vi "Driver Init.vi"(8 "error in (no error)":errorcluster, 11 "SimSyA in":refnum<class "SimSyA.lvclass">) -> (0 "error out":errorcluster, 3 "SimSyA out":refnum<class "SimSyA.lvclass">)   [LabVIEW 2014, in "SimSyA.lvlib" / "SimSyA.lvclass"]
uses:
  SimSyA.lvclass
  SimSyA.lvclass/SimSyA.ctl
  DriverMasterSync/build/DriverMasterSync.lvlibp/Modules/HAL/DriverMasterSync/DriverMasterSyncClass/DriverMasterSync.lvclass
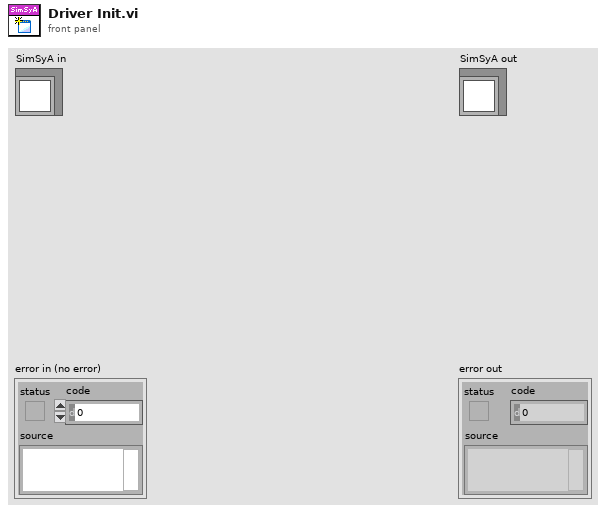
[diagram p1: front panel]
types:
  T1 = typedef "DriverMasterSync.lvlibp/HAL Config Data.ctl" = cluster{"HWSync Index":u32, "Driver Name":string, "Channel Mask":u64}
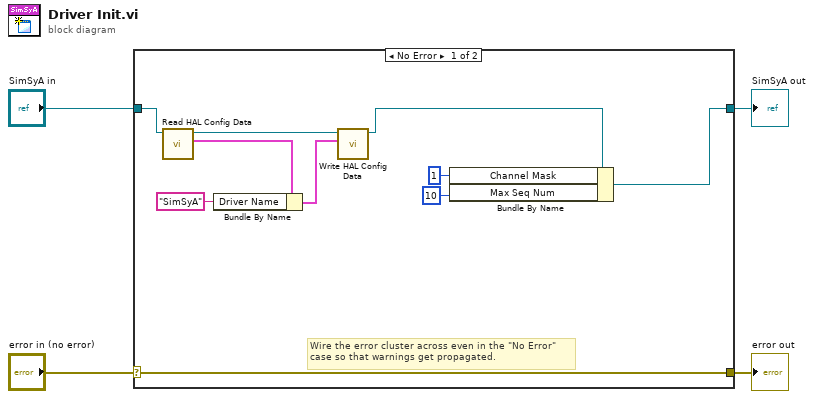
[diagram p0: block diagram]
diagram:
  n1 = case shown="No Error" "error in (no error)" {
    selector: "error in (no error)" -> [w14 w16]
    tunnel: [w14 w16] -> w3
    tunnel: [w13 w15] -> w1
    tunnel: "SimSyA in" -> [w9 w15]
    frame No Error {
      # "Wire the error cluster across even in the \"No Error\"\ncase so that warnings get propagated."
      n2 = call "Read HAL Config Data.vi"("DriverMasterSync in"=w9) -> ("HAL Config Data"=w7:T1, "DriverMasterSync out"=w8:refnum<class "SimSyA.lvclass">)  [unwired: 8 in, 1 out]
      n3 = Bundle By Name(cluster=w7, "Driver Name"="SimSyA") -> (w6:T1)
      n4 = call "Write HAL Config Data.vi"("HAL Config Data"=w6, "DriverMasterSync in"=w8) -> ("DriverMasterSync out"=w10:refnum<class "SimSyA.lvclass">)  [unwired: 8 in, 1 out]
      n5 = Bundle By Name(cluster=w10, "Channel Mask"=u64 1 ("Config Data.Channel Mask"), "Max Seq Num"=u64 10 ("Config Data.Max Seq Num")) -> (w13:refnum<class "SimSyA.lvclass">)
    }
    frame Error {
    }
  }
  "error out" <- w3
  "SimSyA out" <- w1
